vi "Start PES.vi"(0 "Server .py Path":path, 1 "Cmd Line Mode":T1, 2 "port":u16, 5 "Python Executable":path, 11 "Error In":errorcluster) -> (15 "Error Out":errorcluster)   [LabVIEW 2019, in "OPI.lvclass"]
uses:
  OPI.lvclass
  Typedefs/Cmd Line Mode.ctl
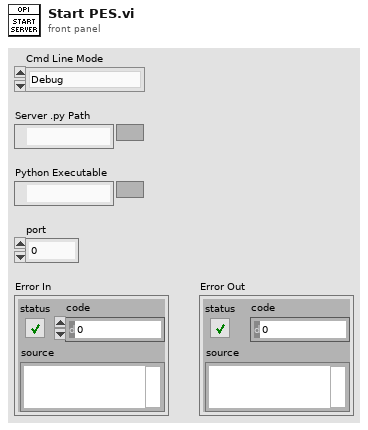
[diagram p1: front panel]
types:
  T1 = typedef "OPI.lvclass/Cmd Line Mode.ctl" = enum16{"Debug", "Hidden"}
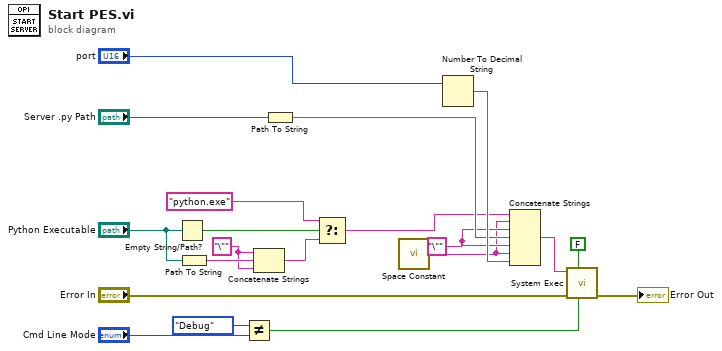
[diagram p0: block diagram]
diagram:
  w1 = "\"" ("string")
  w5 = "\"" ("string")
  n1 = Empty String/Path?(string/path="Python Executable") -> (empty?=w8:bool)
  n2 = Path To String(path="Python Executable") -> (string=w3:string)
  n3 = Not Equal?(x=Cmd_Line_Mode."Debug", y="Cmd Line Mode") -> (x != y?=w12:bool)
  n4 = Concatenate Strings(w1, w3, w1) -> (w2:string)
  n5 = Path To String(path="Server .py Path") -> (string=w14:string)
  n6 = Select(t="python.exe" ("name or relative path"), s=w8, f=w2) -> (s? t:f=w6:string)
  n7 = call <vilib>:"Space Constant.vi"() -> ("String"=w4:string)
  n8 = Number To Decimal String(number="port") -> (decimal integer string=w19:string)  [unwired: 1 in]
  n9 = Concatenate Strings(w6, w4, w5, w14, w5, w4, w19) -> (w15:string)
  n10 = call <vilib>:"System Exec.vi"("run minimized? (F)"=w12, "wait until completion? (T)"=FALSE, "error in (no error)"="Error In", "command line"=w15) -> ("error out"=→"Error Out":errorcluster)  [unwired: 4 in, 3 out]
